vi "AttackerNormalVSS.vi"(9 "balls":T7[](array[typedef]), 10 "IA State":T1={"our_robots"=[], "enemy_robots"=[], "balls"=[], "geometry"={"line_width"=0, "field_length"=0, "field_width"=0, "boundary_width"=0, "referee_width"=0, "goal_width"=0, "goal_depth"=0, "goal_wall_width"=0, "center_circle_radius"=0, "defense_radius"=0, "defense_stretch"=0, "free_kick_from_defense_dist"=0, "penalty_spot_from_field_line_dist"=0, "penalty_line_from_spot_dist"=0}, "IA Judge"={"stage"="", "command"="", "our_goalie_id"=0.0, "enemy_goalie_id"=0.0, "command enum"=enum."Halt", "Time"=enum."Azul"}, "Received Timestamp"=timestamp(0 s since 1904-01-01), "Events"={"Touch"=FALSE, "Ball out"=FALSE, "id touch"=0.0, "Ball out of \nVision"=FALSE, "Ball inside \nGoalie area"=FALSE, "Robot not responding"=FALSE, "Robots responding status"=[1.0, 1.0, 1.0, 1.0, 1.0, 1.0], "Enemy Ball \nPossession"=FALSE, "Pass State"=FALSE, "id end of pass"=0.0, "Kick"=FALSE, "Id ini Possession"=0.0, "Ball Possesion"=FALSE, "Id Possesion"=0.0, "Direct Kick"=FALSE, "2nd Strk Ativo"=FALSE}}, 11 "Robot in":T2={"id"=0, "function"=enum."Attacker", "x"=0.0, "y"=0.0, "orientation"=0.0, "v_tangent"=0.0, "v_normal"=0.0, "v_ang"=0.0, "kick_x"=0.0, "kick_z"=0.0, "dribble"=FALSE, "Timestamp"=timestamp(0 s since 1904-01-01), "estimatives"={"est_v_tangent"=0.0, "est_v_normal"=0.0, "est_vx"=0.0, "est_vy"=0.0, "Pos Robot Est"=[]}, "dest_x_kick"=0.0, "dest_y_kick"=0.0, "Gap Coord"=[], "States"=enum."Pass", "Path "=[], "Path  Smooth"=[], "Dest"=[]}) -> (3 "Robot out":T2={"id"=0, "function"=enum."Attacker", "x"=0.0, "y"=0.0, "orientation"=0.0, "v_tangent"=0.0, "v_normal"=0.0, "v_ang"=0.0, "kick_x"=0.0, "kick_z"=0.0, "dribble"=FALSE, "Timestamp"=timestamp(0 s since 1904-01-01), "estimatives"={"est_v_tangent"=0.0, "est_v_normal"=0.0, "est_vx"=0.0, "est_vy"=0.0, "Pos Robot Est"=[]}, "dest_x_kick"=0.0, "dest_y_kick"=0.0, "Gap Coord"=[], "States"=enum."Pass", "Path "=[], "Path  Smooth"=[], "Dest"=[]})   [LabVIEW 2018]
uses:
  Core/AI Robot.ctl
  Intel/Functions Enum.ctl
  RoboIME/VSS git/VSS/Intel/AttackerStates.ctl
  Path Planning/RRT/PathDests.ctl
  Path Planning/RRT/PathDest.ctl
  Core/AI Ball.ctl
  Core/AI Input.ctl
  Core/Field Size.ctl
  Core/AI Judge.ctl
  Intel/Command Enum.ctl
  Util/Events/Events.ctl
  <vilib>/Analysis/_algsub.llb/Real Vector Norm.vi
  <vilib>/Analysis/NI_AALPro.lvlib
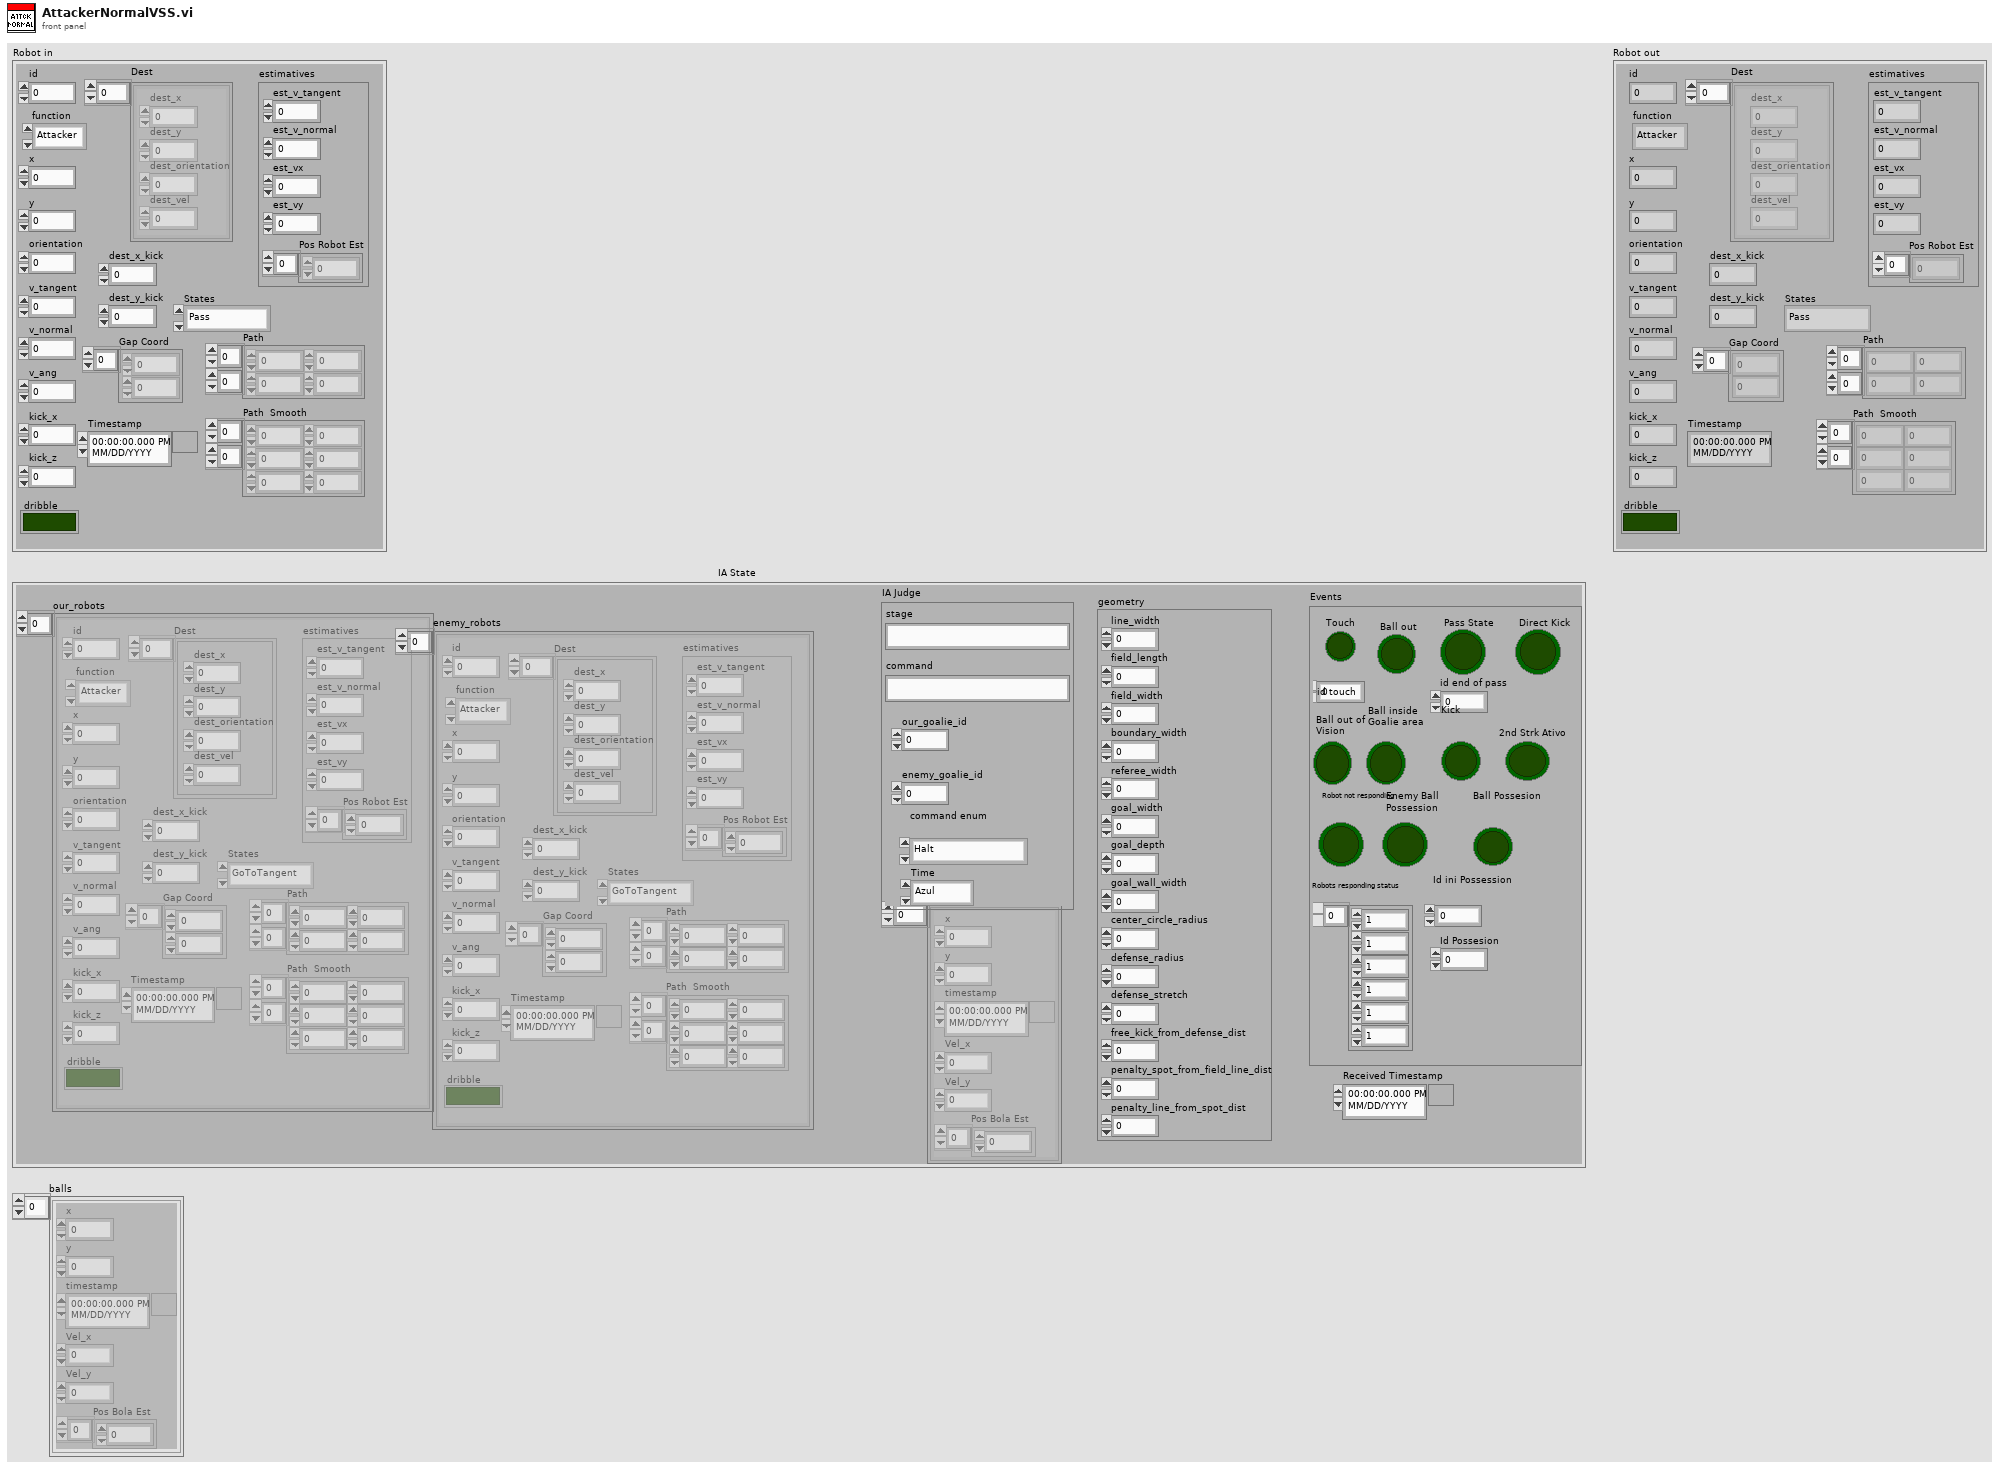
[diagram p1: front panel]
types:
  T1 = typedef "AI Input.ctl" = cluster{"our_robots":T2[], "enemy_robots":T2[], "balls":T7[], "geometry":T8, "IA Judge":T9, "Received Timestamp":timestamp, "Events":T11}
  T2 = typedef "AI Robot.ctl" = cluster{"id":u32, "function":T3, "x":dbl, "y":dbl, "orientation":dbl, "v_tangent":dbl, "v_normal":dbl, "v_ang":dbl, "kick_x":dbl, "kick_z":dbl, "dribble":bool, "Timestamp":timestamp, "estimatives":cluster{"est_v_tangent":dbl, "est_v_normal":dbl, "est_vx":dbl, "est_vy":dbl, "Pos Robot Est":dbl[]}, "dest_x_kick":dbl, "dest_y_kick":dbl, "Gap Coord":dbl[], "States":T4, "Path ":dbl[][], "Path  Smooth":dbl[][], "Dest":T5}
  T3 = typedef "Functions Enum.ctl" = enum16{"2nd Striker", "Attacker", "Goalie", "Defender", "Striker", "Goto 0", "Dummy", "Kicker", "ZigZag 0", "ZigZag 1", "ZigZag 2", "ZigZag 3", "ZigZag 4", "ZigZag 5", "ZigZag 6", "ZigZag 7", "ZigZag 8", ""}
  T4 = typedef "AttackerStates.ctl" = enum16{"Pass", "GoToTangent", "BallGetting", "GoToKick", "Rotate anti-clockwise", "Rotate Clockwise", ""}
  T5 = typedef "PathDests.ctl" = T6[]
  T6 = typedef "PathDest.ctl" = cluster{"dest_x":dbl, "dest_y":dbl, "dest_orientation":dbl, "dest_vel":dbl}
  T7 = typedef "AI Ball.ctl" = cluster{"x":dbl, "y":dbl, "timestamp":timestamp, "Vel_x":dbl, "Vel_y":dbl, "Pos Bola Est":dbl[]}
  T8 = typedef "Field Size.ctl" = cluster{"line_width":u32, "field_length":u32, "field_width":u32, "boundary_width":u32, "referee_width":u32, "goal_width":u32, "goal_depth":u32, "goal_wall_width":u32, "center_circle_radius":u32, "defense_radius":u32, "defense_stretch":u32, "free_kick_from_defense_dist":u32, "penalty_spot_from_field_line_dist":u32, "penalty_line_from_spot_dist":u32}
  T9 = typedef "AI Judge.ctl" = cluster{"stage":string, "command":string, "our_goalie_id":dbl, "enemy_goalie_id":dbl, "command enum":T10, "Time":enum16{"Azul", "Amarelo"}}
  T10 = typedef "Command Enum.ctl" = enum16{"Halt", "Stop", "Force Start", "PKA Normal Start", "Prepare Kickoff Ally", "PKE Normal Start", "Prepare Kickoff Enemy", "Prepare Penalty Ally", "PPA Normal Start", "Prepare Penalty Enemy", "PPE Normal Start", "Direct Free Enemy", "Direct Free Ally", "Indirect Free Enemy", "Indirect Free Ally", "Timeout Enemy", "Timeout Ally", "Goal Enemy", "Goal Ally", "Ball Placement Enemy", "Ball Placement Ally", "Normal Half Time", "Extra Time Break", "Extra Half Time", "None", "Post Game"}
  T11 = typedef "Events.ctl" = cluster{"Touch":bool, "Ball out":bool, "id touch":dbl, "Ball out of \nVision":bool, "Ball inside \nGoalie area":bool, "Robot not responding":bool, "Robots responding status":dbl[], "Enemy Ball \nPossession":bool, "Pass State":bool, "id end of pass":dbl, "Kick":bool, "Id ini Possession":dbl, "Ball Possesion":bool, "Id Possesion":dbl, "Direct Kick":bool, "2nd Strk Ativo":bool}
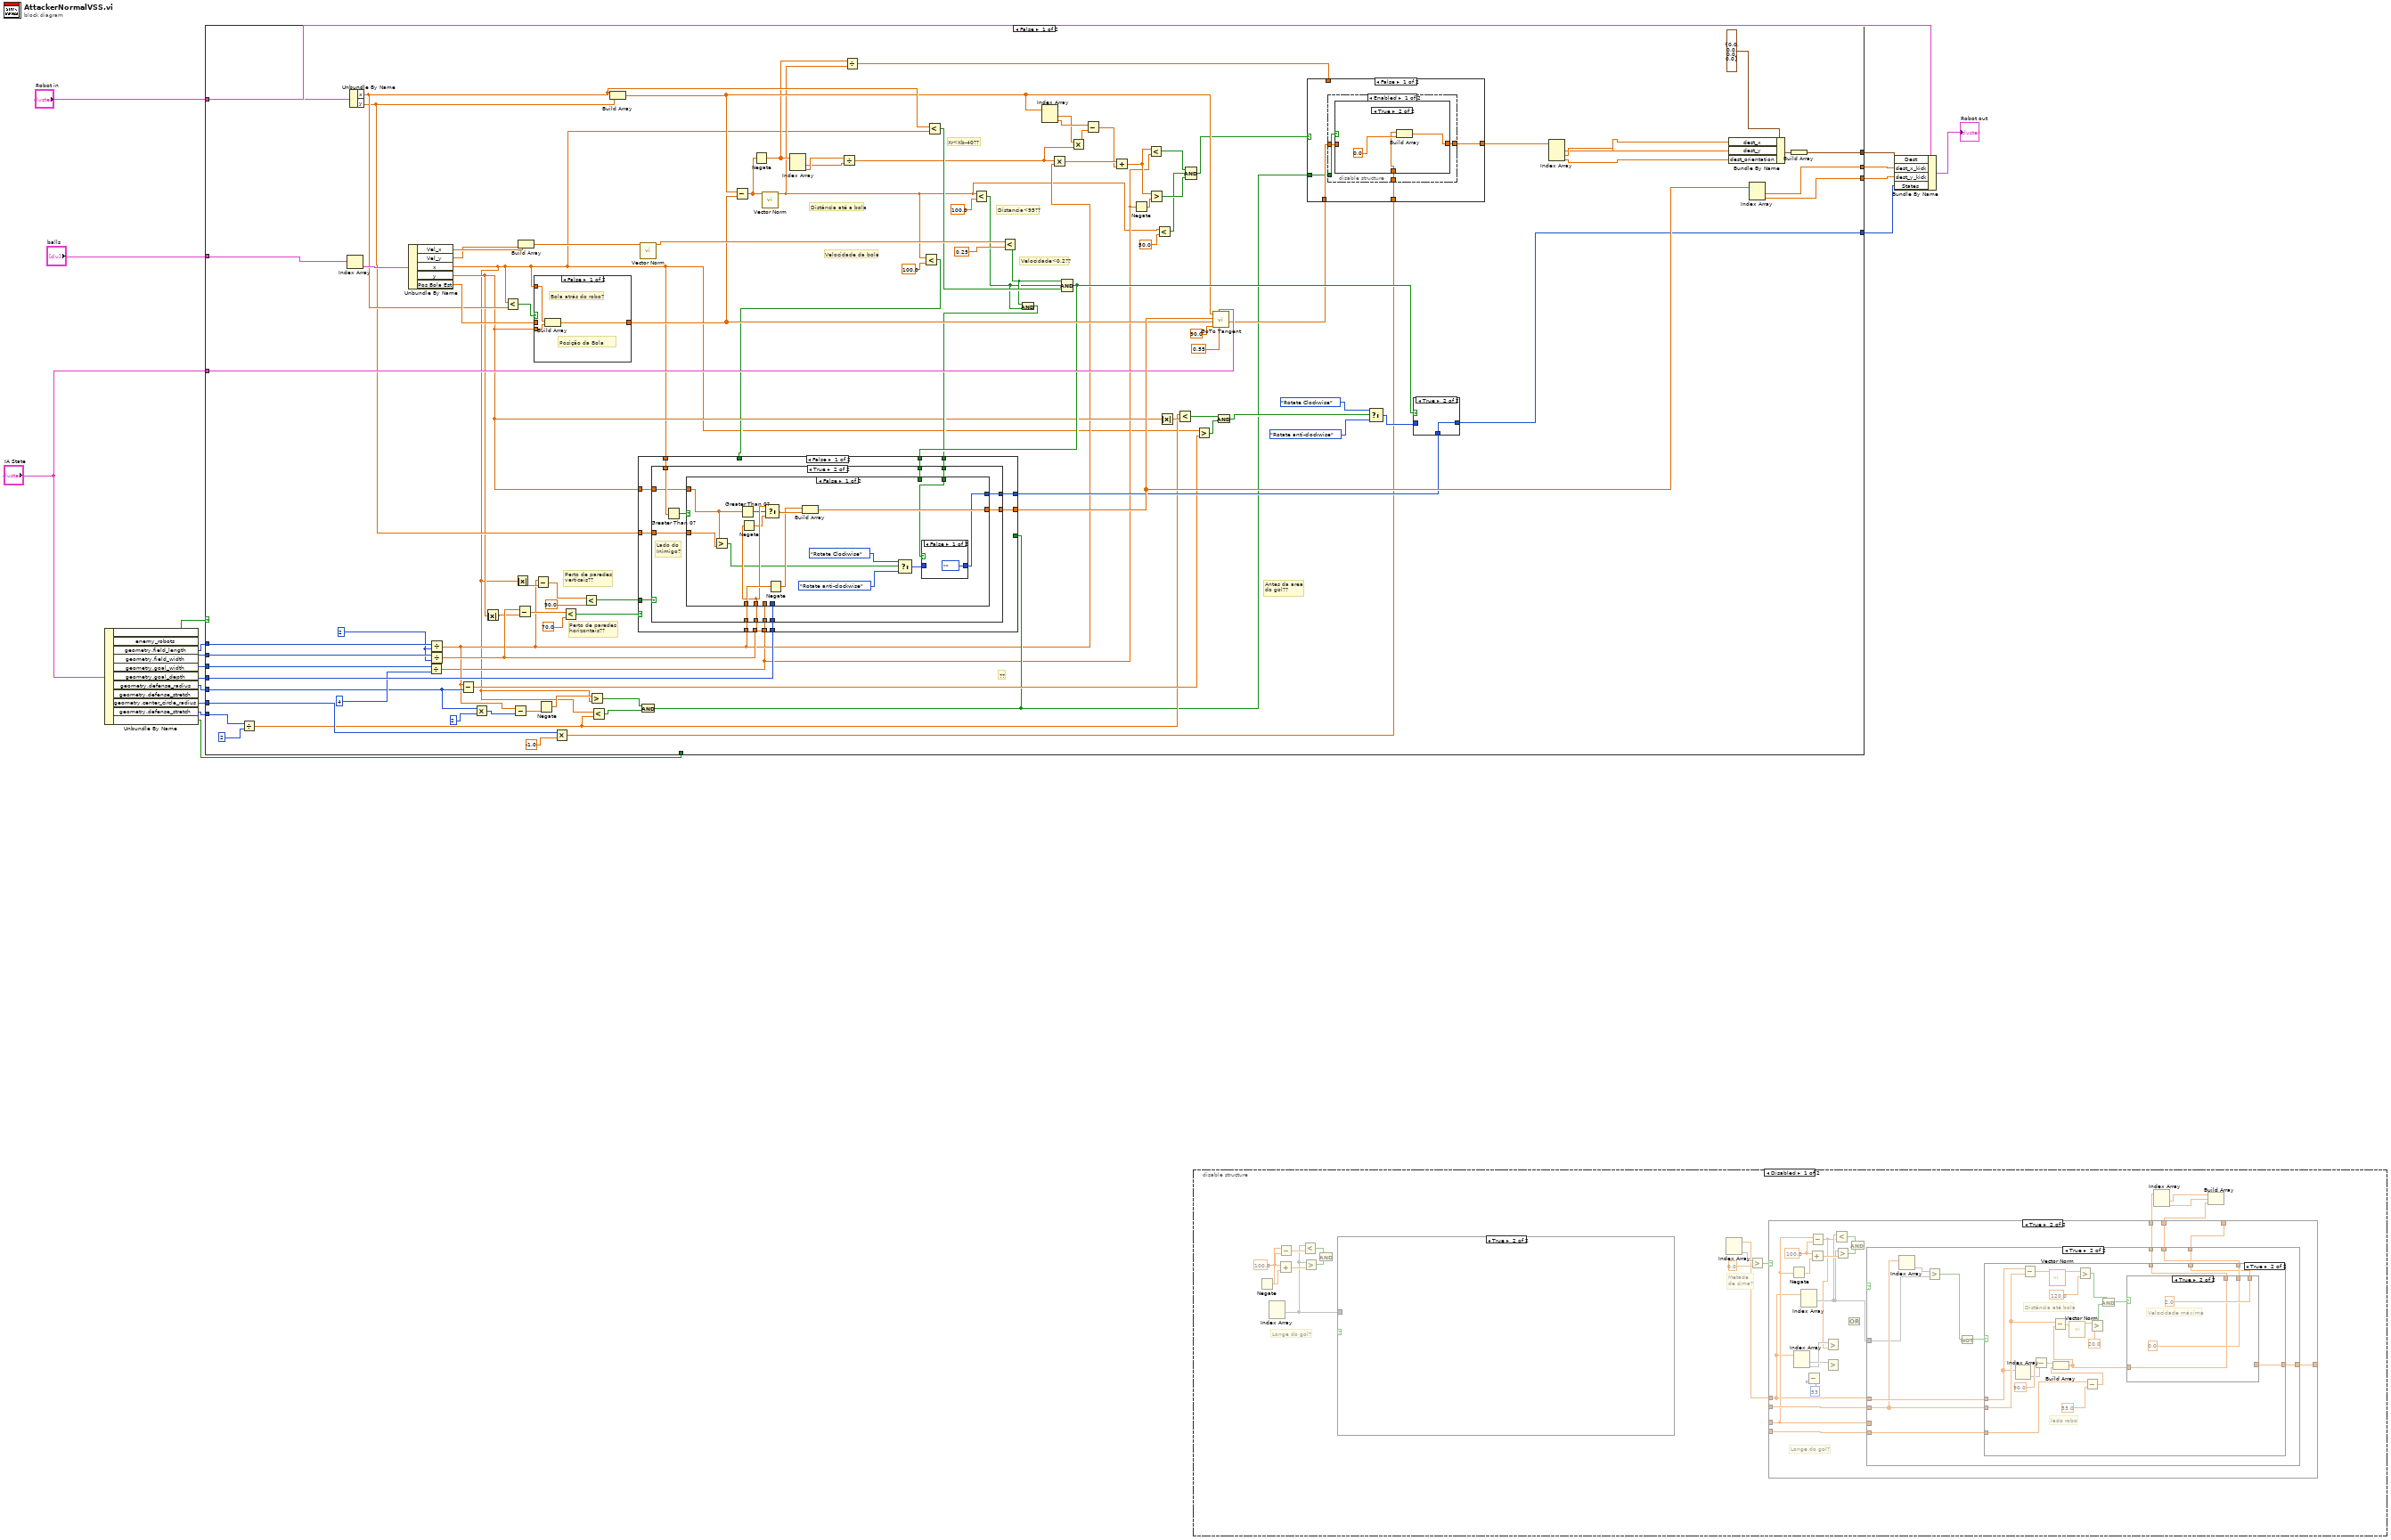
[diagram p0: block diagram]
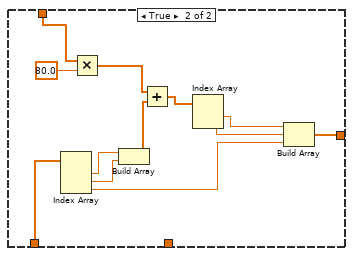
[diagram p4: hidden frame]
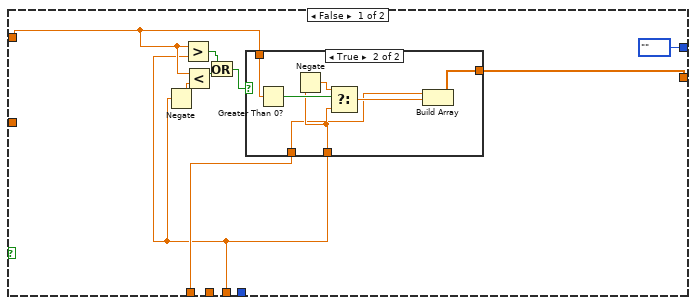
[diagram p7: hidden frame]
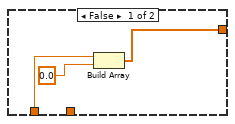
[diagram p8: hidden frame]
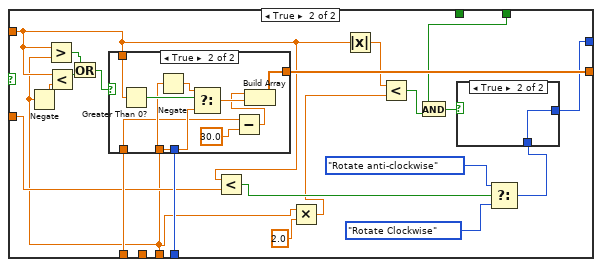
[diagram p10: hidden frame]
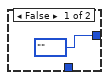
[diagram p11: hidden frame]
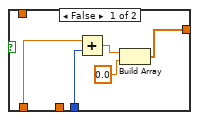
[diagram p12: hidden frame]
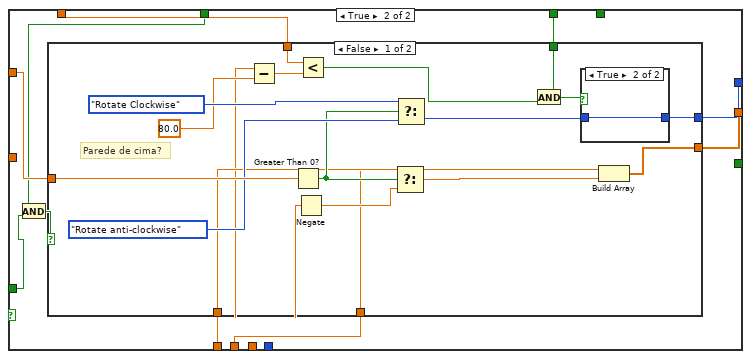
[diagram p13: hidden frame]
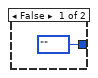
[diagram p14: hidden frame]
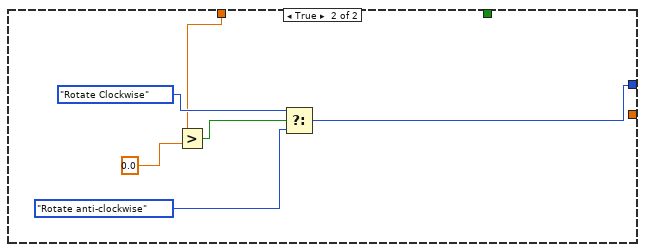
[diagram p15: hidden frame]
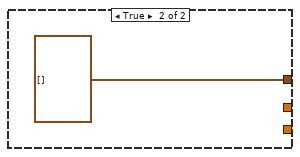
[diagram p16: hidden frame]
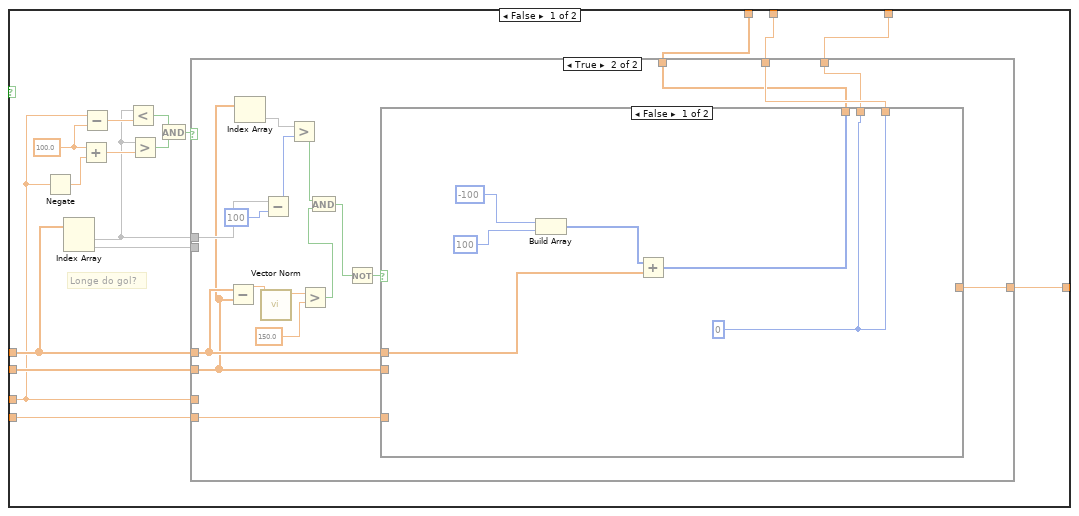
[diagram p17: hidden frame]
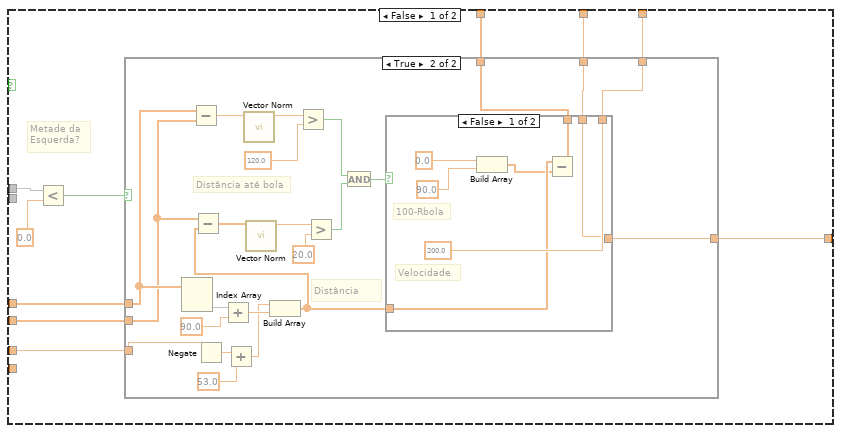
[diagram p18: hidden frame]
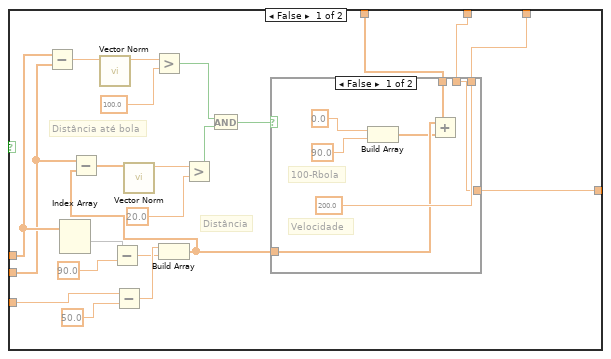
[diagram p19: hidden frame]
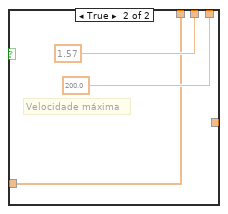
[diagram p20: hidden frame]
diagram:
  n1 = Unbundle By Name("IA State") -> ("Events.Ball out of \nVision"=w3:bool, "geometry.field_length"=w12:u32, "geometry.field_width"=w13:u32, "geometry.goal_width"=w15:u32, "geometry.goal_depth"=w6:u32, "geometry.defense_radius"=w4:u32, "geometry.center_circle_radius"=w1:u32, "geometry.defense_stretch"=w5:u32, "Events.Ball inside \nGoalie area"=w2:bool)  [unwired: 2 out]
  n2 = case shown="False" w3 {
    tunnel: [w115 _] -> w17
    tunnel: [w114 _] -> w16
    tunnel: w15 -> [w112 _]
    tunnel: "IA State" -> [w111 _]
    tunnel: w13 -> [w107 _]
    tunnel: w12 -> [w106 _]
    tunnel: "Robot in" -> [w105 _]
    tunnel: "balls" -> [w104 _]
    tunnel: [w101 T6[] []] -> w9
    tunnel: [w100 _] -> w7
    tunnel: w6 -> [w99 _]
    tunnel: w5 -> [w98 _]
    tunnel: w4 -> [w59 _]
    tunnel: w2 -> [_ _]
    tunnel: w1 -> [w53 _]
    frame False {
      w93 = u32 2 ("y")
      # "Antes da area \ndo gol??"
      # "??"
      # "Perto de paredes \nverticais??"
      # "Perto de paredes \nhorizontais??"
      # "Velocidade<0,2??"
      # "Distancia<95??"
      # "Xr<Xb-40??"
      # "Velocidade da bola"
      # "Distância até a bola"
      n3 = Divide(x=w98, y=u32 2) -> (x/y=w49:dbl)
      n4 = Index Array(array=w104) -> (element=w96:T7)  [unwired: 1 in]
      n5 = Unbundle By Name(w105) -> ("x"=w76:dbl, "y"=w63:dbl)
      n6 = Unbundle By Name(w96) -> ("Vel_x"=w86:dbl, "Vel_y"=w85:dbl, "x"=w18:dbl, "y"=w56:dbl, "Pos Bola Est"=w77:dbl[])
      n7 = Divide(x=w112, y=u32 4) -> (x/y=w27:dbl)
      n8 = Divide(x=w106, y=w93) -> (x/y=w37:dbl)
      n9 = Divide(x=w107, y=w93) -> (x/y=w80:dbl)
      n10 = Subtract(x=w37, y=w59) -> (x-y=w67:dbl)
      n11 = Multiply(x=w59, y=u32 2) -> (x*y=w58:u32)
      n12 = Absolute Value(x=w56) -> (abs(x)=w48:dbl)
      n13 = Less?(x=w18, y=w76) -> (x < y?=w79:bool)
      n14 = Subtract(x=w37, y=w58) -> (x-y=w57:dbl)
      n15 = Absolute Value(x=w18) -> (abs(x)=w92:dbl)
      n16 = Subtract(x=w80, y=w48) -> (x-y=w90:dbl)
      n17 = Build Array(w86, w85) -> (w84:dbl[])
      n18 = case shown="False" w79 {
        tunnel: [w143 w146] -> w78
        tunnel: w77 -> [_ w146]
        tunnel: w18 -> [w145 _]
        tunnel: w56 -> [w144 _]
        frame False {
          # "Bola atrás do robo?"
          # "Posição da Bola"
          n19 = Build Array(w145, w144) -> (w143:dbl[])
        }
        frame True {
          # "Posição futura da bola"
          # "Bola atrás do robo?"
        }
      }
      n20 = Subtract(x=w37, y=w92) -> (x-y=w91:dbl)
      n21 = Negate(x=w57) -> (-x=w55:dbl)
      n22 = Multiply(x=w53, y=-1.0) -> (x*y=w50:dbl)
      n23 = Less?(x=w90, y=70.0) -> (x < y?=w89:bool)
      n24 = Less?(x=w91, y=90.0) -> (x < y?=w88:bool)
      n25 = Greater?(x=w55, y=w18) -> (0:w46:bool)
      n26 = Less?(x=w18, y=w49) -> (x < y?=w47:bool)
      n27 = Build Array(w76, w63) -> (w36:dbl[])
      n28 = call-poly <vilib>:"Vector Norm.vi"("Input Vector"=w84) -> ("norm"=w82:dbl)  [unwired: 9 in, 1 out]
      n29 = And(x=w46, y=w47) -> (x .and. y?=w45:bool)
      n30 = Subtract(x=w36, y=w78) -> (x-y=w40:dbl[])
      n31 = Negate(x=w40) -> (-x=w21:dbl[])
      n32 = call-poly <vilib>:"Vector Norm.vi"("Input Vector"=w40) -> ("norm"=w20:dbl)  [unwired: 9 in, 1 out]
      n33 = Index Array(array=w21) -> (element #1=w38:dbl, element #2=w39:dbl)  [unwired: 2 in]
      n34 = Divide(x=w39, y=w38) -> (x/y=w32:dbl)
      n35 = Divide(x=w21, y=w20) -> (x/y=w19:dbl[])
      n36 = Less?(x=w20, y=100.0) -> (x < y?=w41:bool)
      n37 = Less?(x=w76, y=w18) -> (x < y?=w75:bool)
      n38 = Less?(x=w20, y=100.0) -> (x < y?=w43:bool)
      n39 = Less?(x=w82, y=0.25) -> (x < y?=w62:bool)
      n40 = And(x=w62, y=w43) -> (x .and. y?=w61:bool)
      n41 = Index Array(array=w36) -> (element #1=w33:dbl, element #2=w35:dbl)  [unwired: 2 in]
      n42 = Multiply(x=w32, y=w37) -> (x*y=w34:dbl)
      n43 = Compound Arithmetic op=AND(w62, w43, w75) -> (w70:bool)
      n44 = case shown="False" w89 {
        tunnel: w56 -> [w155 w252]
        tunnel: w80 -> [_ w246]
        tunnel: [w154 w251] -> w113
        tunnel: w88 -> [w157 w244]
        tunnel: w18 -> [w156 w248]
        tunnel: w37 -> [w153 w247]
        tunnel: w27 -> [w149 _]
        tunnel: w70 -> [w152 w249]
        tunnel: [w151 w250] -> w69
        tunnel: w99 -> [w150 _]
        tunnel: w63 -> [w148 _]
        tunnel: w61 -> [w147 _]
        tunnel: w45 -> [_ _]
        tunnel: w41 -> [_ w243]
        frame False {
          n45 = case shown="True" w157 {
            tunnel: w156 -> [_ w187]
            tunnel: w155 -> [w164 w186]
            tunnel: [w165 w185] -> w154
            tunnel: w153 -> [w166 w184]
            tunnel: w152 -> [_ w183]
            tunnel: [AttackerStates."" ("States") w182] -> w151
            tunnel: w150 -> [_ w181]
            tunnel: w149 -> [_ w180]
            tunnel: w149 -> [w162 w179]
            tunnel: w148 -> [_ w178]
            tunnel: w147 -> [_ w177]
            frame False {
              n46 = Negate(x=w162) -> (-x=w161:dbl)
              n47 = Greater?(x=w164, y=w162) -> (0:w158:bool)
              n48 = Less?(x=w164, y=w161) -> (x < y?=w159:bool)
              n49 = Or(x=w158, y=w159) -> (x .or. y?=w160:bool)
              n50 = case shown="True" w160 {
                tunnel: w166 -> [w168 w171]
                tunnel: [w169 w170] -> w165
                tunnel: w164 -> [_ w175]
                tunnel: w162 -> [_ w173]
                frame False {
                  n51 = Build Array(w168, 0.0 ("element")) -> (w169:dbl[])
                }
                frame True {
                  n52 = Greater Than 0?(x=w175) -> (x > 0?=w176:bool)
                  n53 = Negate(x=w173) -> (-x=w174:dbl)
                  n54 = Select(t=w174, s=w176, f=w173) -> (s? t:f=w172:dbl)
                  n55 = Build Array(w171, w172) -> (w170:dbl[])
                }
              }
            }
            frame True {
              # "Lado do\nInimigo?"
              n56 = Greater Than 0?(x=w187) -> (x > 0?=w188:bool)
              n57 = case shown="False" w188 {
                tunnel: w186 -> [w199 w217]
                tunnel: [w203 w221] -> w185
                tunnel: w184 -> [w201 w222]
                tunnel: w183 -> [_ _]
                tunnel: [w202 w212] -> w182
                tunnel: w181 -> [_ w220]
                tunnel: w180 -> [w200 _]
                tunnel: w179 -> [_ w207]
                tunnel: w178 -> [w198 w216]
                tunnel: w177 -> [w197 w209]
                frame False {
                  n58 = Greater?(x=w199, y=w198) -> (0:w189:bool)
                  n59 = Greater Than 0?(x=w199) -> (x > 0?=w192:bool)
                  n60 = Negate(x=w200) -> (-x=w196:dbl)
                  n61 = Select(t=w200, s=w192, f=w196) -> (s? t:f=w195:dbl)
                  n62 = Negate(x=w201) -> (-x=w194:dbl)
                  n63 = Build Array(w194, w195) -> (w203:dbl[])
                  n64 = Select(t=AttackerStates."Rotate Clockwise" ("States"), s=w189, f=AttackerStates."Rotate anti-clockwise" ("States")) -> (s? t:f=w190:T4)
                  n65 = case shown="False" w197 {
                    tunnel: [AttackerStates."" ("States") w205] -> w202
                    tunnel: w190 -> [_ w205]
                    frame False {
                    }
                    frame True {
                    }
                  }
                }
                frame True {
                  n66 = Negate(x=w207) -> (-x=w226:dbl)
                  n67 = Greater?(x=w217, y=w207) -> (0:w223:bool)
                  n68 = Less?(x=w217, y=w226) -> (x < y?=w224:bool)
                  n69 = Or(x=w223, y=w224) -> (x .or. y?=w225:bool)
                  n70 = case shown="True" w225 {
                    tunnel: w222 -> [w229 w234]
                    tunnel: [w232 w237] -> w221
                    tunnel: w217 -> [_ w241]
                    tunnel: w207 -> [_ w239]
                    tunnel: w220 -> [w230 _]
                    frame False {
                      n71 = Add(x=w229, y=w230) -> (x+y=w231:dbl)
                      n72 = Build Array(w231, 0.0 ("element")) -> (w232:dbl[])
                    }
                    frame True {
                      n73 = Greater Than 0?(x=w241) -> (x > 0?=w242:bool)
                      n74 = Negate(x=w239) -> (-x=w240:dbl)
                      n75 = Select(t=w240, s=w242, f=w239) -> (s? t:f=w238:dbl)
                      n76 = Subtract(x=w234, y=30.0) -> (x-y=w235:dbl)
                      n77 = Build Array(w235, w238) -> (w237:dbl[])
                    }
                  }
                  n78 = Less?(x=w217, y=w216) -> (x < y?=w215:bool)
                  n79 = Multiply(x=w207, y=2.0) -> (x*y=w206:dbl)
                  n80 = Absolute Value(x=w217) -> (abs(x)=w219:dbl)
                  n81 = Less?(x=w219, y=w206) -> (x < y?=w210:bool)
                  n82 = And(x=w209, y=w210) -> (x .and. y?=w211:bool)
                  n83 = Select(t=AttackerStates."Rotate anti-clockwise" ("States"), s=w215, f=AttackerStates."Rotate Clockwise" ("States")) -> (s? t:f=w218:T4)
                  n84 = case shown="True" w211 {
                    tunnel: w218 -> [_ w228]
                    tunnel: [AttackerStates."" ("States") w228] -> w212
                    frame False {
                    }
                    frame True {
                    }
                  }
                }
              }
            }
          }
        }
        frame True {
          n85 = And(x=w243, y=w244) -> (x .and. y?=w245:bool)
          n86 = case shown="False" w245 {
            tunnel: w252 -> [w269 _]
            tunnel: [w266 _] -> w251
            tunnel: [w263 w272] -> w250
            tunnel: w249 -> [w261 _]
            tunnel: w248 -> [w260 w273]
            tunnel: w247 -> [w254 _]
            tunnel: w246 -> [w253 _]
            frame False {
              # "Parede de cima?"
              n87 = Subtract(x=w253, y=80.0) -> (x-y=w259:dbl)
              n88 = Greater Than 0?(x=w269) -> (x > 0?=w262:bool)
              n89 = Negate(x=w253) -> (-x=w268:dbl)
              n90 = Less?(x=w260, y=w259) -> (x < y?=w256:bool)
              n91 = Select(t=w253, s=w262, f=w268) -> (s? t:f=w267:dbl)
              n92 = Select(t=AttackerStates."Rotate Clockwise" ("States"), s=w262, f=AttackerStates."Rotate anti-clockwise" ("States")) -> (s? t:f=w257:T4)
              n93 = And(x=w261, y=w256) -> (x .and. y?=w255:bool)
              n94 = case shown="True" w255 {
                tunnel: w257 -> [_ w271]
                tunnel: [AttackerStates."" ("States") w271] -> w263
                frame False {
                }
                frame True {
                }
              }
              n95 = Build Array(w254, w267) -> (w266:dbl[])
            }
            frame True {
              n96 = Greater?(x=w273, y=0.0) -> (0:w274:bool)
              n97 = Select(t=AttackerStates."Rotate Clockwise" ("States"), s=w274, f=AttackerStates."Rotate anti-clockwise" ("States")) -> (s? t:f=w272:T4)
            }
          }
        }
      }
      n98 = Multiply(x=w33, y=w32) -> (x*y=w31:dbl)
      n99 = Subtract(x=w35, y=w31) -> (x-y=w30:dbl)
      n100 = Add(x=w34, y=w30) -> (x+y=w29:dbl)
      n101 = Negate(x=w27) -> (-x=w28:dbl)
      n102 = Less?(x=w29, y=w27) -> (x < y?=w26:bool)
      n103 = Greater?(x=w29, y=w28) -> (0:w25:bool)
      n104 = Less?(x=w20, y=50.0) -> (x < y?=w23:bool)
      n105 = Absolute Value(x=w56) -> (abs(x)=w68:dbl)
      n106 = Less?(x=w49, y=w68) -> (x < y?=w66:bool)
      n107 = Compound Arithmetic op=AND(w26, w23, w25) -> (w22:bool)
      n108 = Greater?(x=w18, y=w67) -> (0:w65:bool)
      n109 = call "GoTo Tangent.vi"("Cone de chute"=0.55, "IA State Input in"=w111, "distance between ball and robot"=90.0, "Ball"=w78, "Target"=w113, "R"=w36) -> ("Destination"=w52:dbl[])  [unwired: 4 in, 1 out]
      n110 = And(x=w66, y=w65) -> (x .and. y?=w64:bool)
      n111 = case shown="False" w22 {
        tunnel: w52 -> [w119 w140]
        tunnel: [w118 w129] -> w51
        tunnel: w50 -> [w117 _]
        tunnel: w45 -> [w116 _]
        tunnel: w19 -> [_ w138]
        frame False {
          n112 = disable-structure shown="Enabled" {
            disable-tunnel: w119 -> [w123 w128]
            disable-tunnel: [w122 w128] -> w118
            disable-tunnel: w117 -> [w121 _]
            disable-tunnel: w116 -> [w120 _]
            frame Enabled {
              n113 = case shown="True" w120 {
                tunnel: [w124 w127] -> w122
                tunnel: w123 -> [w124 _]
                tunnel: w121 -> [_ w125]
                frame False {
                }
                frame True {
                  n114 = Build Array(w125, 0.0 ("y")) -> (w127:dbl[])
                }
              }
            }
            frame Disabled {
            }
          }
        }
        frame True {
          n115 = Index Array(array=w140) -> (element #1=w135:dbl, element #2=w134:dbl, element #3=w130:dbl)  [unwired: 3 in]
          n116 = Multiply(x=w138, y=80.0) -> (x*y=w137:dbl[])
          n117 = Build Array(w135, w134) -> (w136:dbl[])
          n118 = Add(x=w137, y=w136) -> (x+y=w133:dbl[])
          n119 = Index Array(array=w133) -> (element #1=w132:dbl, element #2=w131:dbl)  [unwired: 2 in]
          n120 = Build Array(w132, w131, w130) -> (w129:dbl[])
        }
      }
      n121 = Select(t=AttackerStates."Rotate Clockwise" ("States"), s=w64, f=AttackerStates."Rotate anti-clockwise" ("States")) -> (s? t:f=w71:T4)
      n122 = case shown="True" w70 {
        tunnel: [w141 w142] -> w100
        tunnel: w71 -> [_ _]
        tunnel: w69 -> [w141 w142]
        frame False {
        }
        frame True {
        }
      }
      n123 = Index Array(array=w51) -> (element #1=w109:dbl, element #2=w110:dbl, element #3=w108:dbl)  [unwired: 3 in]
      n124 = Bundle By Name(cluster=T6 {"dest_x"=0.0, "dest_y"=0.0, "dest_orientation"=0.0, "dest_vel"=0.0} ("element"), "dest_x"=w109, "dest_y"=w110, "dest_orientation"=w108) -> (w102:T6)
      n125 = Index Array(array=w113) -> (element #1=w114:dbl, element #2=w115:dbl)  [unwired: 2 in]
      n126 = Build Array(w102) -> (w101:T6[])
    }
    frame True {
    }
  }
  n127 = disable-structure shown="Disabled" {
    frame Disabled {
      w299 = 100.0
      # "Metade \nde cima?"
      # "Longe do gol?"
      n128 = Index Array() -> (array=w294:dbl[], element #1=w293)  [unwired: 2 in, 1 out]
      n129 = Subtract(y=w299) -> (x=w292:dbl, x-y=w298:dbl)
      n130 = Negate(x=w292) -> (-x=w300:dbl)
      n131 = Add(x=w299, y=w300) -> (x+y=w297:dbl)
      n132 = Less?(x=w293, y=w298) -> (x < y?=w295:bool)
      n133 = Greater?(x=w293, y=w297) -> (0:w296:bool)
      n134 = And(x=w295, y=w296) -> ()  [unwired: 1 out]
      n135 = case shown="True" {
        selector: _ -> [_ _]
        tunnel: w293 -> [_ _]
        frame False {
        }
        frame True {
        }
      }
      n136 = Index Array(array=w288) -> (element #2=w290)  [unwired: 2 in, 1 out]
      n137 = Greater?(x=w290, y=0.0) -> (0:w289:bool)
      n138 = case shown="True" w289 {
        tunnel: [w317 w457] -> _
        tunnel: [w316 w456] -> w281
        tunnel: [w312 w453] -> w288
        tunnel: [w315 w460] -> w287
        tunnel: [w304 w459] -> w285
        tunnel: [w306 w461] -> w286
        tunnel: [w303 w458] -> w284
        tunnel: [w302 w455] -> w279
        frame False {
          w313 = 100.0
          # "Longe do gol?"
          n139 = Negate(x=w304) -> (-x=w314:dbl)
          n140 = Index Array(array=w312) -> (element #1=w305, element #2=w301)  [unwired: 2 in]
          n141 = Add(x=w313, y=w314) -> (x+y=w310:dbl)
          n142 = Subtract(x=w304, y=w313) -> (x-y=w311:dbl)
          n143 = Less?(x=w305, y=w311) -> (x < y?=w308:bool)
          n144 = Greater?(x=w305, y=w310) -> (0:w309:bool)
          n145 = And(x=w308, y=w309) -> (x .and. y?=w307:bool)
          n146 = case shown="True" w307 {
            tunnel: [w327 w393] -> w317
            tunnel: [w326 w395] -> w316
            tunnel: w312 -> [w322 w407]
            tunnel: w315 -> [w321 w400]
            tunnel: w306 -> [_ w410]
            tunnel: w305 -> [w324 w401]
            tunnel: w304 -> [w320 _]
            tunnel: [w319 w394] -> w303
            tunnel: w302 -> [w318 w409]
            tunnel: w301 -> [_ _]
            frame False {
              # "Metade da \nEsquerda?"
              n147 = Less?(x=w324, y=0.0) -> (x < y?=w323:bool)
              n148 = case shown="True" w323 {
                tunnel: [w349 w382] -> w327
                tunnel: [w348 w381] -> w326
                tunnel: w322 -> [w341 w374]
                tunnel: w321 -> [w334 w366]
                tunnel: w320 -> [w338 w371]
                tunnel: [w329 w361] -> w319
                tunnel: w318 -> [w328 w360]
                frame False {
                  # "Distância até bola"
                  # "Distância"
                  n149 = Subtract(x=w341, y=w334) -> (x-y=w344:dbl)
                  n150 = Index Array(array=w341) -> (element #2=w340)  [unwired: 2 in, 1 out]
                  n151 = call-poly <vilib>:"Vector Norm.vi"("Input Vector"=w344) -> ("norm"=w343:dbl)  [unwired: 9 in, 1 out]
                  n152 = Subtract(x=w340, y=90.0) -> (x-y=w335:dbl)
                  n153 = Subtract(x=w338, y=50.0) -> (x-y=w336:dbl)
                  n154 = Greater?(x=w343, y=100.0) -> (0:w332:bool)
                  n155 = Build Array(w336, w335) -> (w333:dbl[])
                  n156 = Subtract(x=w334, y=w333) -> (x-y=w345:dbl[])
                  n157 = call-poly <vilib>:"Vector Norm.vi"("Input Vector"=w345) -> ("norm"=w347:dbl)  [unwired: 9 in, 1 out]
                  n158 = Greater?(x=w347, y=20.0) -> (0:w331:bool)
                  n159 = And(x=w332, y=w331) -> (x .and. y?=w330:bool)
                  n160 = case shown="False" w330 {
                    tunnel: [200.0 200.0] -> w349
                    tunnel: [w350 1.57] -> w348
                    tunnel: w333 -> [w353 w357]
                    tunnel: [w351 w357] -> w329
                    tunnel: w328 -> [w350 _]
                    frame False {
                      # "100-Rbola"
                      # "Velocidade"
                      n161 = Build Array(0.0, 90.0) -> (w352:dbl[])
                      n162 = Add(x=w353, y=w352) -> (x+y=w351:dbl[])
                    }
                    frame True {
                      # "Velocidade máxima"
                    }
                  }
                }
                frame True {
                  # "Distância até bola"
                  # "Distância"
                  n163 = Index Array(array=w374) -> (element #2=w372)  [unwired: 2 in, 1 out]
                  n164 = Subtract(x=w374, y=w366) -> (x-y=w377:dbl)
                  n165 = Negate(x=w371) -> (-x=w370:dbl)
                  n166 = Add(x=w372, y=90.0) -> (x+y=w368:dbl)
                  n167 = Add(x=w370, y=53.0) -> (x+y=w367:dbl)
                  n168 = call-poly <vilib>:"Vector Norm.vi"("Input Vector"=w377) -> ("norm"=w376:dbl)  [unwired: 9 in, 1 out]
                  n169 = Build Array(w367, w368) -> (w365:dbl[])
                  n170 = Subtract(x=w366, y=w365) -> (x-y=w378:dbl[])
                  n171 = call-poly <vilib>:"Vector Norm.vi"("Input Vector"=w378) -> ("norm"=w380:dbl)  [unwired: 9 in, 1 out]
                  n172 = Greater?(x=w376, y=120.0) -> (0:w363:bool)
                  n173 = Greater?(x=w380, y=20.0) -> (0:w362:bool)
                  n174 = And(x=w363, y=w362) -> (x .and. y?=w364:bool)
                  n175 = case shown="False" w364 {
                    tunnel: [200.0 200.0] -> w382
                    tunnel: [w383 1.57] -> w381
                    tunnel: w365 -> [w385 w390]
                    tunnel: [w386 w390] -> w361
                    tunnel: w360 -> [w383 _]
                    frame False {
                      # "100-Rbola"
                      # "Velocidade"
                      n176 = Build Array(0.0, 90.0) -> (w384:dbl[])
                      n177 = Subtract(x=w385, y=w384) -> (x-y=w386:dbl[])
                    }
                    frame True {
                      # "Velocidade máxima"
                    }
                  }
                }
              }
            }
            frame True {
              n178 = Subtract(x=w407, y=w400) -> (x-y=w406:dbl)
              n179 = Index Array(array=w400) -> (element=w399)  [unwired: 1 in]
              n180 = call-poly <vilib>:"Vector Norm.vi"("Input Vector"=w406) -> ("norm"=w405:dbl)  [unwired: 9 in, 1 out]
              n181 = Subtract(x=w401, y=100) -> (x-y=w398:i32)
              n182 = Greater?(x=w399, y=w398) -> (0:w408:bool)
              n183 = Greater?(x=w405, y=150.0) -> (0:w397:bool)
              n184 = And(x=w408, y=w397) -> (x .and. y?=w396:bool)
              n185 = Not(x=w396) -> (.not. x?=w403:bool)
              n186 = case shown="False" w403 {
                tunnel: w400 -> [_ w433]
                tunnel: w407 -> [w413 w427]
                tunnel: w410 -> [_ w424]
                tunnel: w409 -> [_ w420]
                tunnel: [w412 w419] -> w394
                tunnel: [w411 w418] -> w395
                tunnel: [w411 w417] -> w393
                frame False {
                  w411 = 0
                  n187 = Build Array(-100, 100) -> (w414:i32[])
                  n188 = Add(x=w414, y=w413) -> (x+y=w412:i32[])
                }
                frame True {
                  # "lado robo"
                  # "Distância até bola"
                  n189 = Index Array(array=w427) -> (element=w428)  [unwired: 1 in]
                  n190 = Subtract(x=w427, y=w433) -> (x-y=w436:dbl)
                  n191 = Subtract(x=w428, y=90.0) -> (x-y=w423:dbl)
                  n192 = Negate(x=w424) -> (-x=w425:dbl)
                  n193 = call-poly <vilib>:"Vector Norm.vi"("Input Vector"=w436) -> ("norm"=w435:dbl)  [unwired: 9 in, 1 out]
                  n194 = Greater?(x=w435, y=120.0) -> (0:w431:bool)
                  n195 = Add(x=w425, y=53.0) -> (x+y=w422:dbl)
                  n196 = Build Array(w423, w422) -> (w421:dbl[])
                  n197 = Subtract(x=w433, y=w421) -> (x-y=w437:dbl[])
                  n198 = call-poly <vilib>:"Vector Norm.vi"("Input Vector"=w437) -> ("norm"=w439:dbl)  [unwired: 9 in, 1 out]
                  n199 = Greater?(x=w439, y=20.0) -> (0:w432:bool)
                  n200 = And(x=w431, y=w432) -> (x .and. y?=w430:bool)
                  n201 = case shown="False" w430 {
                    tunnel: [0.0 2.0] -> w417
                    tunnel: w421 -> [w442 w448]
                    tunnel: [w441 w448] -> w419
                    tunnel: [w440 0.0] -> w418
                    tunnel: w420 -> [w440 _]
                    frame False {
                      # "100-Rbola"
                      # "Velocidade máxima"
                      n202 = Build Array(90.0, 0.0) -> (w443:dbl[])
                      n203 = Add(x=w443, y=w442) -> (x+y=w441:dbl[])
                    }
                    frame True {
                      # "Velocidade máxima"
                    }
                  }
                }
              }
            }
          }
        }
        frame True {
          w466 = 100.0
          # "Longe do gol?"
          n204 = Negate(x=w459) -> (-x=w467:dbl)
          n205 = Index Array(array=w453) -> (element #1=w454, element #2=w452)  [unwired: 2 in]
          n206 = Index Array(array=w453) -> (element #1=w462)  [unwired: 2 in, 1 out]
          n207 = Subtract(y=53) -> ()  [unwired: 1 in, 1 out]
          n208 = Add(x=w466, y=w467) -> (x+y=w465:dbl)
          n209 = Subtract(x=w459, y=w466) -> (x-y=w451:dbl)
          n210 = Greater?(x=w454, y=w451) -> ()  [unwired: 1 out]
          n211 = Greater?(x=w452) -> ()  [unwired: 1 in, 1 out]
          n212 = Less?(x=w462, y=w451) -> (x < y?=w463:bool)
          n213 = Greater?(x=w462, y=w465) -> (0:w464:bool)
          n214 = Or() -> ()  [unwired: 2 in, 1 out]
          n215 = And(x=w463, y=w464) -> ()  [unwired: 1 out]
          n216 = case shown="True" {
            selector: _ -> [_ _]
            tunnel: [w477 w544] -> w456
            tunnel: w453 -> [w473 w549]
            tunnel: w460 -> [w472 w548]
            tunnel: w461 -> [_ w553]
            tunnel: w462 -> [w475 w547]
            tunnel: w459 -> [w471 _]
            tunnel: [w470 w545] -> w458
            tunnel: [w469 w543] -> w457
            tunnel: w455 -> [w468 w552]
            frame False {
              # "Metade da \nEsquerda?"
              n217 = Less?(x=w475, y=0.0) -> (x < y?=w474:bool)
              n218 = case shown="False" w474 {
                tunnel: [w499 w532] -> w477
                tunnel: w473 -> [w492 w525]
                tunnel: w472 -> [w485 w517]
                tunnel: w471 -> [w489 w522]
                tunnel: [w480 w512] -> w470
                tunnel: [w479 w511] -> w469
                tunnel: w468 -> [w478 w510]
                frame False {
                  # "Distância até bola"
                  # "Distância"
                  n219 = Subtract(x=w492, y=w485) -> (x-y=w495:dbl)
                  n220 = Index Array(array=w492) -> (element #2=w491)  [unwired: 2 in, 1 out]
                  n221 = call-poly <vilib>:"Vector Norm.vi"("Input Vector"=w495) -> ("norm"=w494:dbl)  [unwired: 9 in, 1 out]
                  n222 = Add(x=w491, y=90.0) -> (x+y=w486:dbl)
                  n223 = Subtract(x=w489, y=53.0) -> (x-y=w487:dbl)
                  n224 = Greater?(x=w494, y=100.0) -> (0:w483:bool)
                  n225 = Build Array(w487, w486) -> (w484:dbl[])
                  n226 = Subtract(x=w485, y=w484) -> (x-y=w496:dbl[])
                  n227 = call-poly <vilib>:"Vector Norm.vi"("Input Vector"=w496) -> ("norm"=w498:dbl)  [unwired: 9 in, 1 out]
                  n228 = Greater?(x=w498, y=20.0) -> (0:w482:bool)
                  n229 = And(x=w483, y=w482) -> (x .and. y?=w481:bool)
                  n230 = case shown="False" w481 {
                    tunnel: [200.0 2.0] -> w479
                    tunnel: [w500 1.57] -> w499
                    tunnel: w484 -> [w503 w507]
                    tunnel: [w501 w507] -> w480
                    tunnel: w478 -> [w500 _]
                    frame False {
                      # "100-Rbola"
                      # "Velocidade"
                      n231 = Build Array(0.0, 90.0) -> (w502:dbl[])
                      n232 = Subtract(x=w503, y=w502) -> (x-y=w501:dbl[])
                    }
                    frame True {
                      # "Velocidade máxima"
                    }
                  }
                }
                frame True {
                  # "Distância até bola"
                  # "Distância"
                  n233 = Index Array(array=w525) -> (element #2=w523)  [unwired: 2 in, 1 out]
                  n234 = Subtract(x=w525, y=w517) -> (x-y=w528:dbl)
                  n235 = Negate(x=w522) -> (-x=w521:dbl)
                  n236 = Subtract(x=w523, y=90.0) -> (x-y=w519:dbl)
                  n237 = Add(x=w521, y=53.0) -> (x+y=w518:dbl)
                  n238 = call-poly <vilib>:"Vector Norm.vi"("Input Vector"=w528) -> ("norm"=w527:dbl)  [unwired: 9 in, 1 out]
                  n239 = Build Array(w518, w519) -> (w516:dbl[])
                  n240 = Subtract(x=w517, y=w516) -> (x-y=w529:dbl[])
                  n241 = call-poly <vilib>:"Vector Norm.vi"("Input Vector"=w529) -> ("norm"=w531:dbl)  [unwired: 9 in, 1 out]
                  n242 = Greater?(x=w527, y=120.0) -> (0:w514:bool)
                  n243 = Greater?(x=w531, y=20.0) -> (0:w513:bool)
                  n244 = And(x=w514, y=w513) -> (x .and. y?=w515:bool)
                  n245 = case shown="False" w515 {
                    tunnel: [2.0 200.0] -> w511
                    tunnel: [w533 1.57] -> w532
                    tunnel: w516 -> [w536 w540]
                    tunnel: [w534 w540] -> w512
                    tunnel: w510 -> [w533 _]
                    frame False {
                      # "100-Rbola"
                      # "Velocidade"
                      n246 = Build Array(0.0, 90.0) -> (w535:dbl[])
                      n247 = Add(x=w535, y=w536) -> (x+y=w534:dbl[])
                    }
                    frame True {
                      # "Velocidade máxima"
                    }
                  }
                }
              }
            }
            frame True {
              n248 = Index Array(array=w548) -> (element=w550)  [unwired: 1 in]
              n249 = Greater?(x=w550, y=w547) -> (0:w551:bool)
              n250 = Not(x=w551) -> (.not. x?=w546:bool)
              n251 = case shown="True" w546 {
                tunnel: w548 -> [_ w575]
                tunnel: w549 -> [w556 w569]
                tunnel: w553 -> [_ w567]
                tunnel: w552 -> [_ w563]
                tunnel: [w555 w562] -> w545
                tunnel: [w554 w561] -> w544
                tunnel: [w554 w560] -> w543
                frame False {
                  w554 = 0
                  n252 = Build Array(-100, -100) -> (w557:i32[])
                  n253 = Add(x=w557, y=w556) -> (x+y=w555:i32[])
                }
                frame True {
                  # "lado robo"
                  # "Distância até bola"
                  n254 = Index Array(array=w569) -> (element=w570)  [unwired: 1 in]
                  n255 = Subtract(x=w569, y=w575) -> (x-y=w578:dbl)
                  n256 = Subtract(x=w570, y=90.0) -> (x-y=w566:dbl)
                  n257 = call-poly <vilib>:"Vector Norm.vi"("Input Vector"=w578) -> ("norm"=w577:dbl)  [unwired: 9 in, 1 out]
                  n258 = Greater?(x=w577, y=120.0) -> (0:w573:bool)
                  n259 = Subtract(x=w567, y=53.0) -> (x-y=w565:dbl)
                  n260 = Build Array(w566, w565) -> (w564:dbl[])
                  n261 = Subtract(x=w575, y=w564) -> (x-y=w579:dbl[])
                  n262 = call-poly <vilib>:"Vector Norm.vi"("Input Vector"=w579) -> ("norm"=w581:dbl)  [unwired: 9 in, 1 out]
                  n263 = Greater?(x=w581, y=20.0) -> (0:w574:bool)
                  n264 = And(x=w573, y=w574) -> (x .and. y?=w572:bool)
                  n265 = case shown="True" w572 {
                    tunnel: [2.0 2.0] -> w560
                    tunnel: w564 -> [w584 w590]
                    tunnel: [w583 w590] -> w562
                    tunnel: [w582 0.0] -> w561
                    tunnel: w563 -> [w582 _]
                    frame False {
                      # "100-Rbola"
                      # "Velocidade máxima"
                      n266 = Build Array(90.0, 0.0) -> (w585:dbl[])
                      n267 = Add(x=w585, y=w584) -> (x+y=w583:dbl[])
                    }
                    frame True {
                      # "Velocidade máxima"
                    }
                  }
                }
              }
            }
          }
        }
      }
      n268 = Index Array(array=w284) -> (element #1=w283:dbl, element #2=w282:dbl)  [unwired: 2 in]
      n269 = Build Array(w283, w282, w281) -> (w280:dbl[])
    }
    frame Enabled {
    }
  }
  n270 = Bundle By Name(cluster="Robot in", "Dest"=w9, "dest_x_kick"=w16, "dest_y_kick"=w17, "States"=w7) -> (→"Robot out":T2)
